vi "Create.vi"(5 "TestSuite In":refnum<class "TestSuite.lvclass">, 8 "error in (no error)":errorcluster, 10 "Path":path) -> (0 "error out":errorcluster, 3 "TestSuite":refnum<class "TestSuite.lvclass">)   [LabVIEW 2019, in "TestSuite.lvclass"]
uses:
  TestSuite.lvclass
  <vilib>/Utility/error.llb/Error Cluster From Error Code.vi
  <vilib>/ErrorRing/Error Ring.xnode
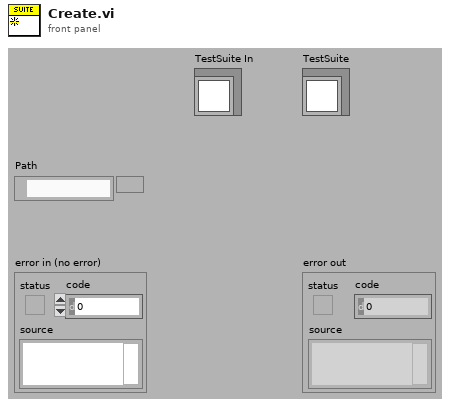
[diagram p1: front panel]
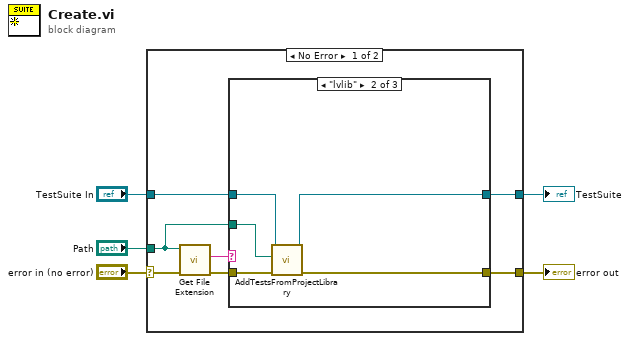
[diagram p0: block diagram]
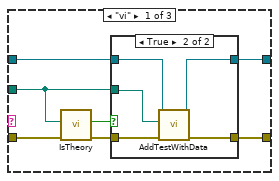
[diagram p2: hidden frame]
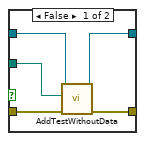
[diagram p3: hidden frame]
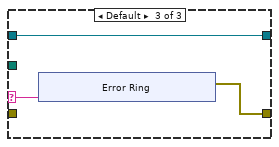
[diagram p4: hidden frame]
diagram:
  n1 = case shown="No Error" "error in (no error)" {
    selector: "error in (no error)" -> [w12 w46]
    tunnel: [w10 w46] -> w4
    tunnel: [w7 w45] -> w2
    tunnel: "TestSuite In" -> [w8 w45]
    tunnel: "Path" -> [w6 _]
    frame No Error {
      n2 = call <vilib>:"Get File Extension.vi"("error in (no error)"=w12, "file"=w6) -> ("error out"=w9:errorcluster, "lowercase file extension"=w11:string)  [unwired: 5 in, 3 out]
      n3 = case shown="\"lvlib\"" w11 {
        selector: w11 -> [_ _ w37]
        tunnel: [w19 w33 w36] -> w10
        tunnel: w9 -> [w16 w34 _]
        tunnel: w8 -> [w18 w32 w35]
        tunnel: [w17 w31 w35] -> w7
        tunnel: w6 -> [w14 w30 _]
        frame "vi" {
          n4 = call "IsTheory.vi"("error in (no error)"=w16, "VI Path"=w14) -> ("error out"=w15:errorcluster, "Is Theory?"=w13:bool)  [unwired: 8 in]
          n5 = case shown="True" w13 {
            tunnel: [w24 w28] -> w19
            tunnel: w18 -> [w23 w26]
            tunnel: [w22 w25] -> w17
            tunnel: w15 -> [w21 w29]
            tunnel: w14 -> [w20 w27]
            frame False {
              n6 = call "AddTestWithoutData.vi"("error in (no error)"=w21, "Path"=w20, "TestSuite in"=w23) -> ("error out"=w24:errorcluster, "TestSuite out"=w22:refnum<class "TestSuite.lvclass">)  [unwired: 7 in]
            }
            frame True {
              n7 = call "AddTestWithData.vi"("error in (no error)"=w29, "Path"=w27, "TestSuite in"=w26) -> ("error out"=w28:errorcluster, "TestSuite out"=w25:refnum<class "TestSuite.lvclass">)  [unwired: 7 in]
            }
          }
        }
        frame "lvlib" {
          n8 = call "AddTestsFromProjectLibrary.vi"("error in (no error)"=w34, "Path"=w30, "TestSuite in"=w32) -> ("error out"=w33:errorcluster, "TestSuite out"=w31:refnum<class "TestSuite.lvclass">)  [unwired: 7 in]
        }
        frame Default {
          n9 = xnode "Error Ring"("parameter 0"=w37) -> ("error out"=w36:errorcluster)
        }
      }
    }
    frame Error {
    }
  }
  "error out" <- w4
  "TestSuite" <- w2
